vi "search first nonzero element (CDB).vi"(10 "Numbers":cdb[](array[numeric])) -> (2 "first nonzero element":cdb)   [LabVIEW 2024, in "NI_AALPro.lvlib"]
uses:
  NI_AALPro.lvlib
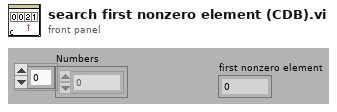
[diagram p1: front panel]
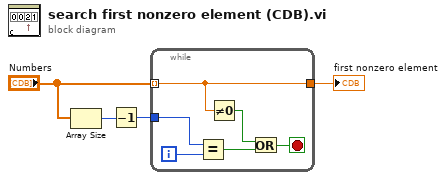
[diagram p0: block diagram]
diagram:
  n1 = Array Size(array="Numbers") -> (size(s)=w2:i32)
  n2 = Decrement(x=w2) -> (x-1=w1:i32)
  n3 = while {
    tunnel: "Numbers" -> [w10] mode=indexing
    tunnel: [w10] -> w4
    tunnel: w1 -> [w9]
    i -> [w8]
    stop <- w5 stop-if-true
    n4 = Equal?(x=w9, y=w8) -> (x = y?=w6:bool)
    n5 = Not Equal To 0?(x=w10) -> (x != 0?=w7:bool)
    n6 = Or(x=w7, y=w6) -> (x .or. y?=w5:bool)
  }
  "first nonzero element" <- w4
